vi "eReadName Multiple Call Loop.vi"() -> (0 "error out":errorcluster)   [LabVIEW 2020]
panel:
  out "Iteration":u32
  out "Value B":dbl format="%.6f"
  in  "Name B":string="AIN0"
  out "Value A":dbl format="%.6f"
  in  "Name A":string="AIN0"
  in  "stop":bool
  in  "Interval [ms]":i32=500
  out "Error String":string
  out "ConnectionType Out":i32
  out "DeviceType Out":i32
  in  "Identifier":string="LJM_idANY"
  in  "ConnectionType":string="LJM_ctANY"
  in  "DeviceType":string="LJM_dtANY"
  # "This VI demonstrates 2 calls to eReadName in\na loop.  The example \"eReadNames Loop.vi\"\ndemonstrates a more efficient techique of\none call to eReadNames rather than multiple\ncalls to eReadName."
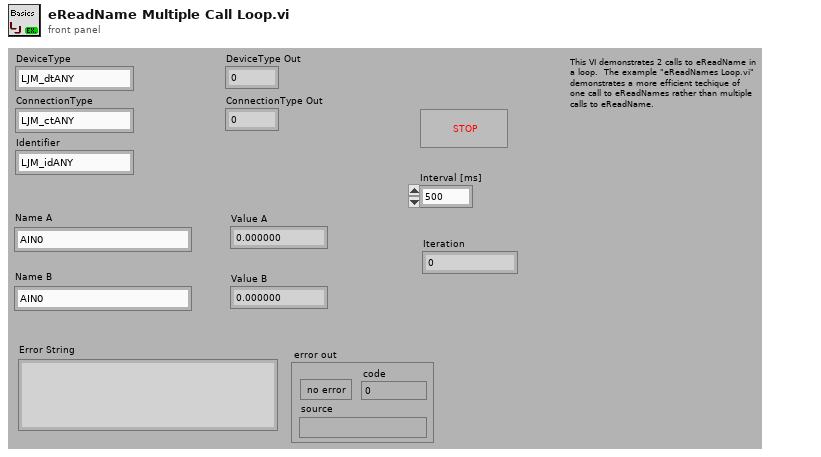
[diagram p1: front panel]
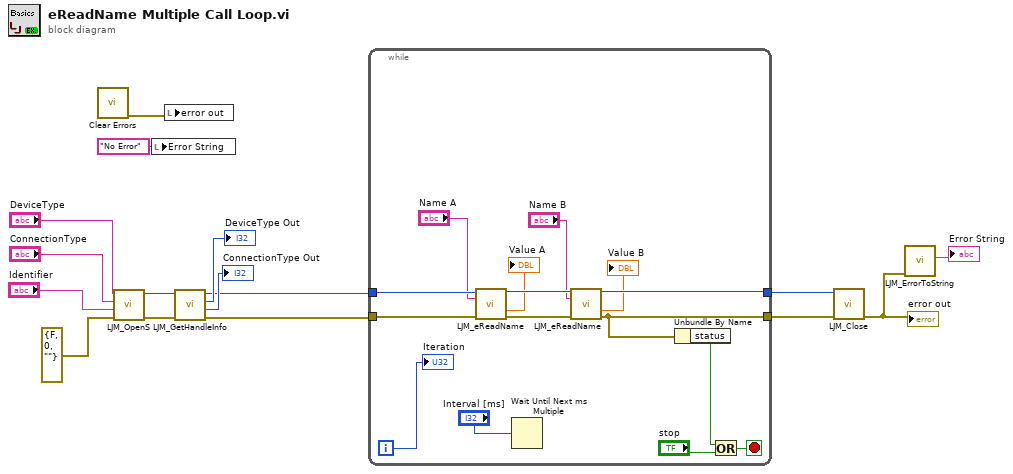
[diagram p0: block diagram]
diagram:
  n1 = call <vilib>:"Clear Errors.vi"() -> ("error out"=w3:errorcluster)  [unwired: 6 in, 1 out]
  n2 = call "LJM_OpenS.vi"("error in"=errorcluster {"status"=FALSE, "code"=0, "source"=""}, "Identifier"="Identifier", "ConnectionType"="ConnectionType", "DeviceType"="DeviceType") -> ("error out"=w16:errorcluster, "Handle"=w15:i32)  [unwired: 6 in]
  n3 = local write "Error String"("No Error" ("Error String")) -> ()
  n4 = local write "error out"(w3) -> ()
  n5 = call "LJM_GetHandleInfo.vi"("error in"=w16, "Handle In"=w15) -> ("error out"=w4:errorcluster, "ConnectionType"=→"ConnectionType Out":i32, "DeviceType"=→"DeviceType Out":i32, "Handle Out"=w5:i32)  [unwired: 2 in, 4 out]
  n6 = while {
    tunnel: w4 -> [w31]
    tunnel: [w24] -> w7
    tunnel: w5 -> [w30]
    tunnel: [w22] -> w6
    i -> [w17]
    stop <- w28 stop-if-true
    n7 = call "LJM_eReadName.vi"("Handle In"=w30, "Name"="Name A", "error in"=w31) -> ("Handle Out"=w23:i32, "Value"=→"Value A":dbl, "error out"=w25:errorcluster)  [unwired: 10 in]
    n8 = Wait Until Next ms Multiple(millisecond multiple="Interval [ms]") -> ()  [unwired: 1 out]
    n9 = call "LJM_eReadName.vi"("Handle In"=w23, "Name"="Name B", "error in"=w25) -> ("Handle Out"=w22:i32, "Value"=→"Value B":dbl, "error out"=w24:errorcluster)  [unwired: 10 in]
    n10 = Unbundle By Name(w24) -> ("status"=w27:bool)
    n11 = Or(x=w27, y="stop") -> (x .or. y?=w28:bool)
    "Iteration" <- w17
  }
  n12 = call "LJM_Close.vi"("error in"=w7, "Handle"=w6) -> ("error out"=w9:errorcluster)  [unwired: 9 in]
  "error out" <- w9
  n13 = call "LJM_ErrorToString.vi"("error in"=w9) -> ("String"=→"Error String":string)  [unwired: 10 in]
